vi "harmonic well.vi"() -> ()   [LabVIEW 2019]
uses:
  <vilib>/eio/EIONode/EIONode.xnode
  <vilib>/rvi/eio/common/nirviEmuTemplateMethod_errors.vi
  <vilib>/rvi/DataTransferAndStorage/Container/XNode/niFpgaContainer.xnode
  <vilib>/rvi/FIFO/Fifo_Resource/nirvififoEmulationRead.vi
  <vilib>/eio/EIOPropertyNode/EIOPropertyNode.xnode
  <vilib>/rvi/eio/common/nirviEmuTemplatePropertyGet_errors.vi
  <vilib>/rvi/eio/common/nirviEmuTemplatePropertyGet_noerrors.vi
  <vilib>/rvi/eio/common/nirviEmuTemplatePropertySet_errors.vi
  <vilib>/rvi/eio/common/nirviEmuTemplatePropertySet_noerrors.vi
  <vilib>/rvi/FIFO/Fifo_Resource/nirvififoEmulationWrite.vi
  <vilib>/rvi/interface/RandomDataEmulation/nirviRandomDataFpgaReadWriteTemplate.vi
panel:
  in  "1/Ycali":sgl
  out "Fy out/Ycorr":sgl
  in  "MobY(px/V)":sgl
  in  "Ymean":sgl
  in  "DY":sgl
  in  "Feedback parameters Y":T1
  in  "Enum":enum8{"No FB", "FB"}(ring)
  in  "MobX(px/V)":sgl
  in  "1/Xcali":sgl
  in  "Feedback parameters":T1
  in  "DX":sgl
  in  "Xmean":sgl
  in  "Frequency":u32=100000
  in  "Triangle wave":T2={"signal offset_X"=5.0, "Scale X"=0.0, "signal offset_Y"=5.0, "Scale Y"=0.0, "Phase Shift"=30}
  out "Fx out/Xcorr":sgl
  in  "Xoffset":sgl
  in  "Yoffset":sgl
  in  "sum_offset":sgl
  in  "Normalize signal":bool=TRUE
  in  "FB Time":u8=5 caption="Feedback loop time"
  out "Saveloop":u32
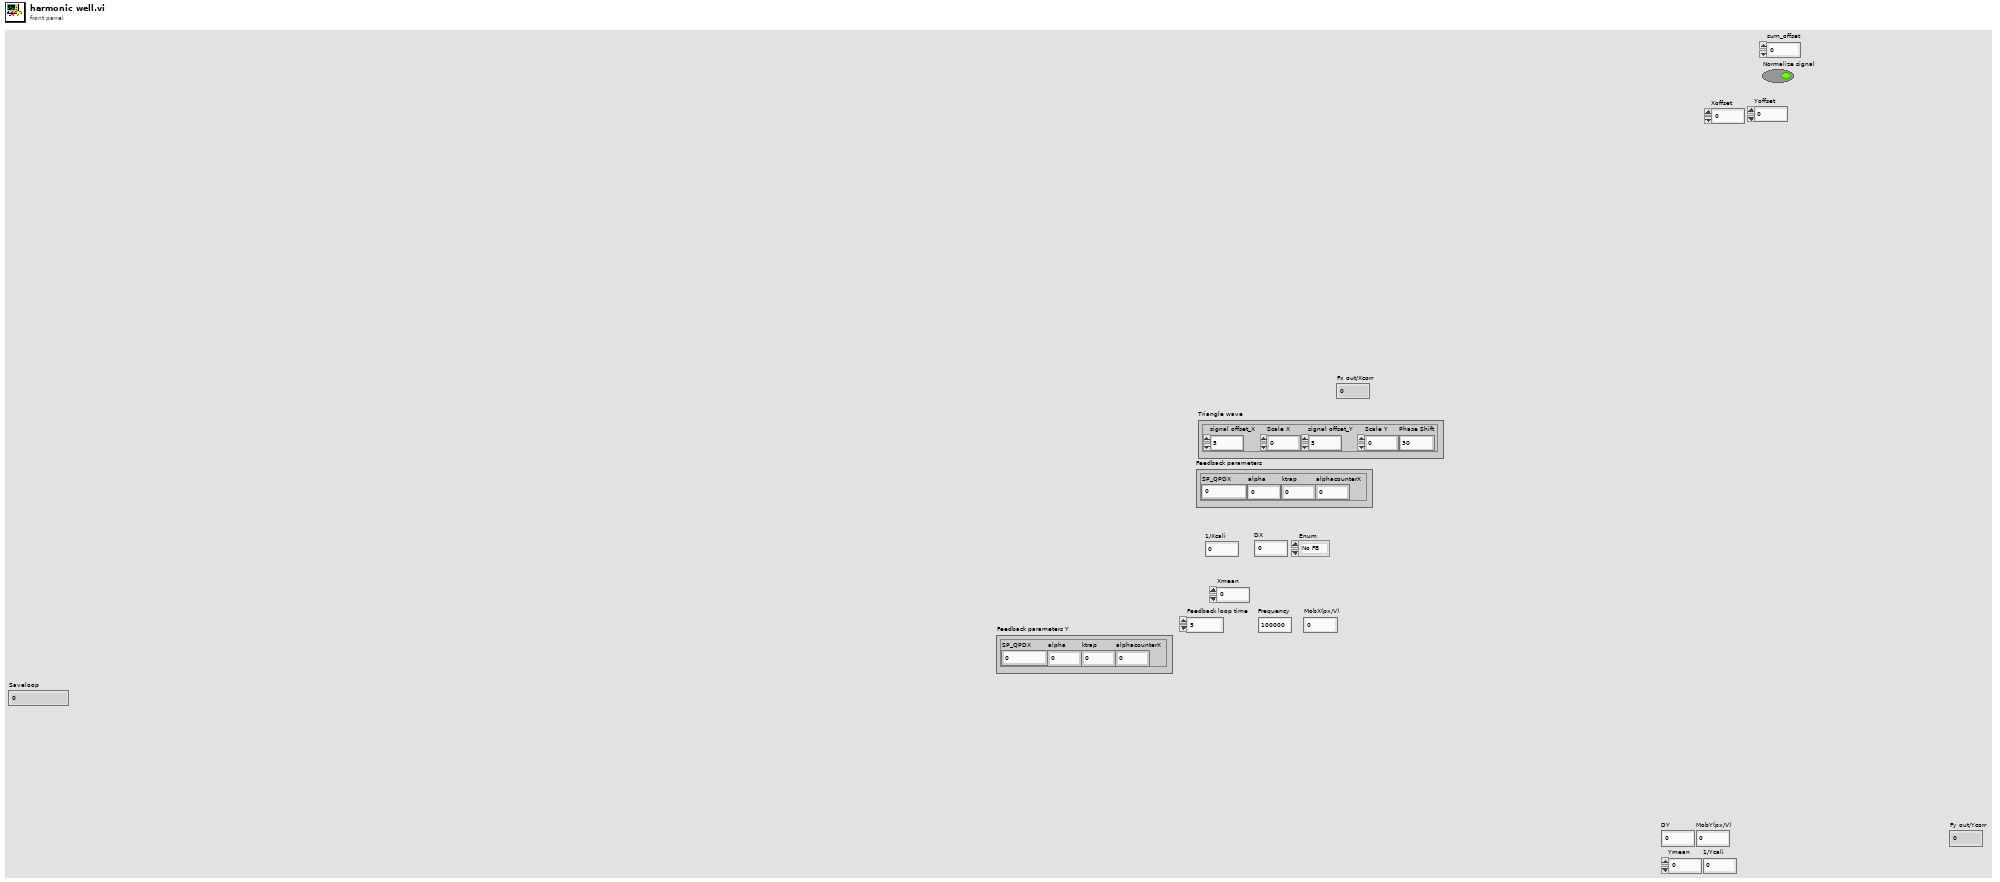
[diagram p1: front panel]
types:
  T1 = cluster{"SP_QPDX":sgl, "alpha":sgl, "ktrap":sgl, "alphacounterX":sgl}
  T2 = cluster{"signal offset_X":sgl, "Scale X":sgl, "signal offset_Y":sgl, "Scale Y":sgl, "Phase Shift":u32}
  T3 = enum8{"+/- 10 V", "+/- 5 V", "+/- 2 V", "+/- 1 V"}
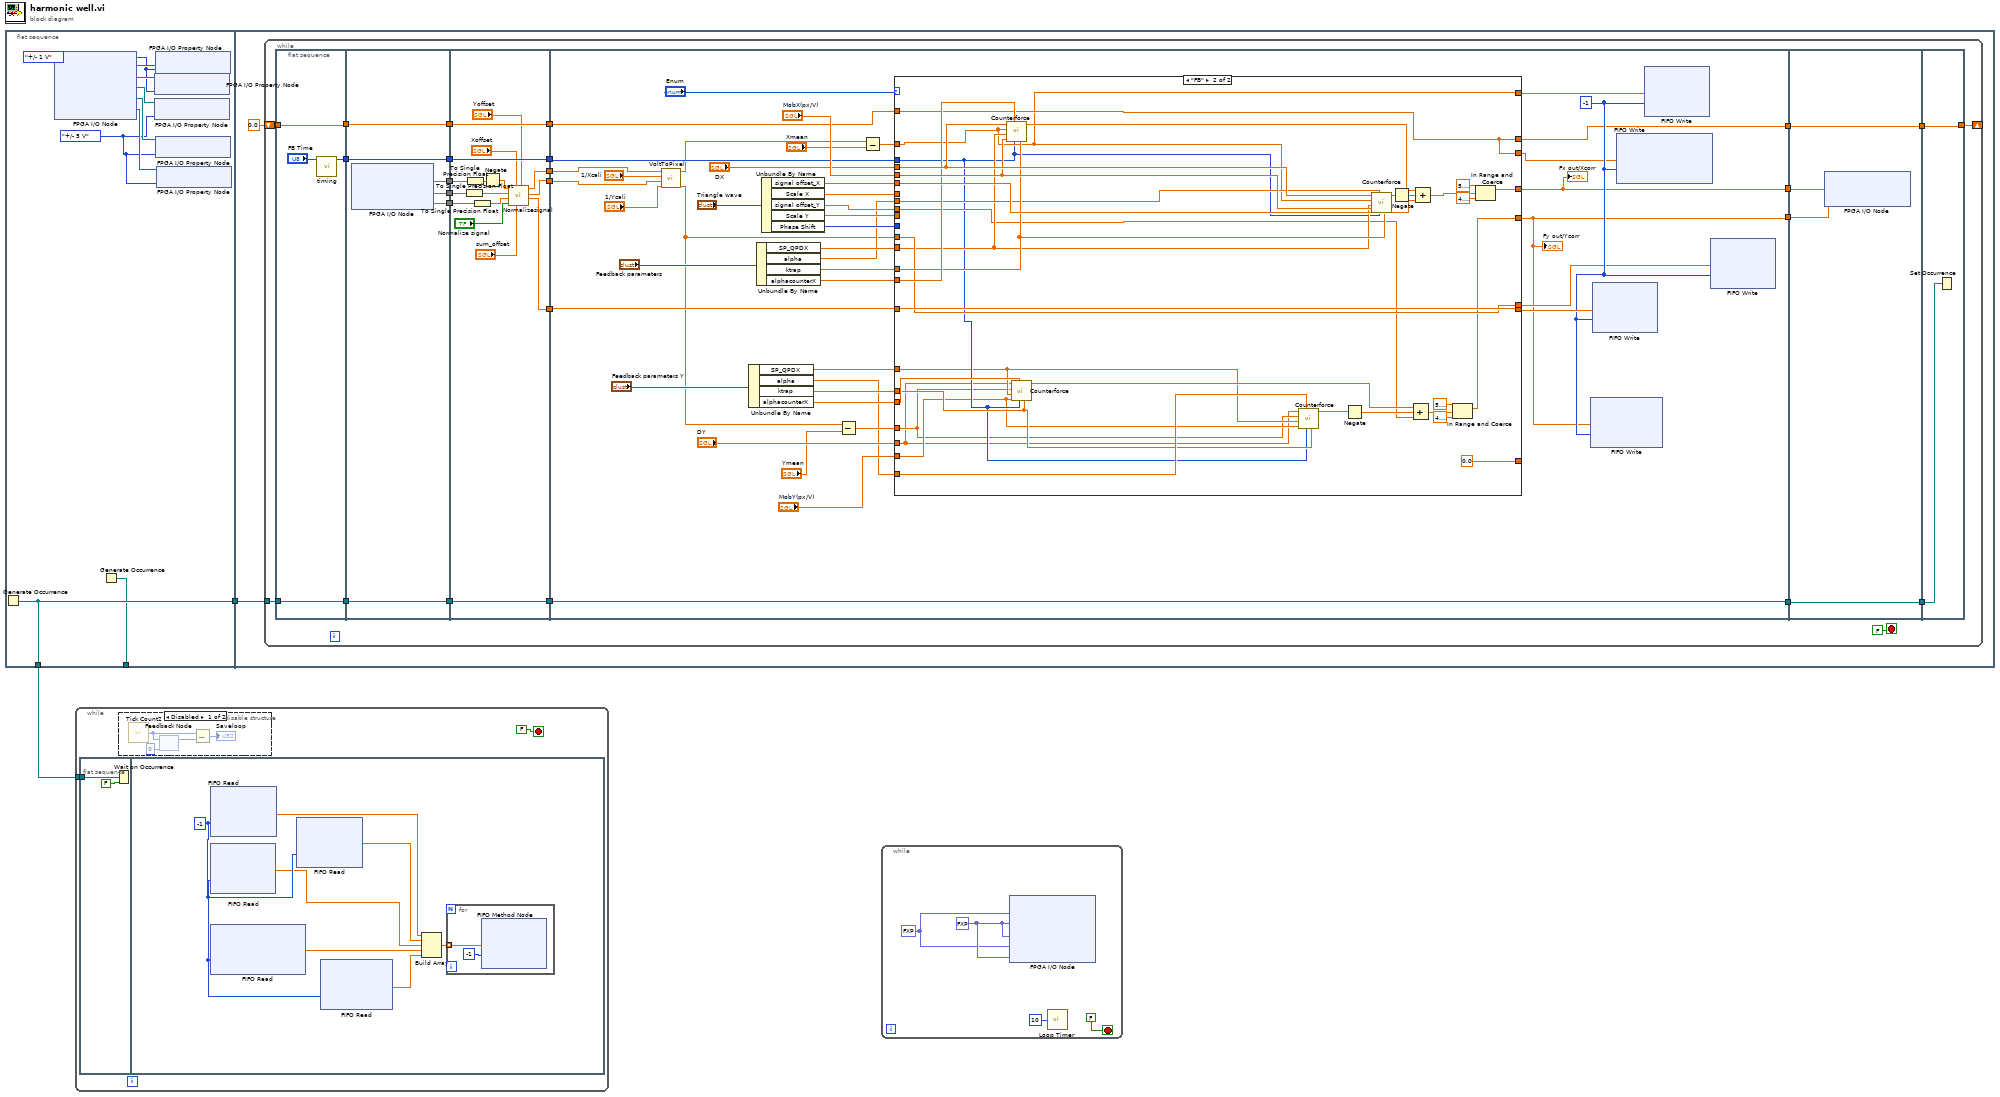
[diagram p0: block diagram]
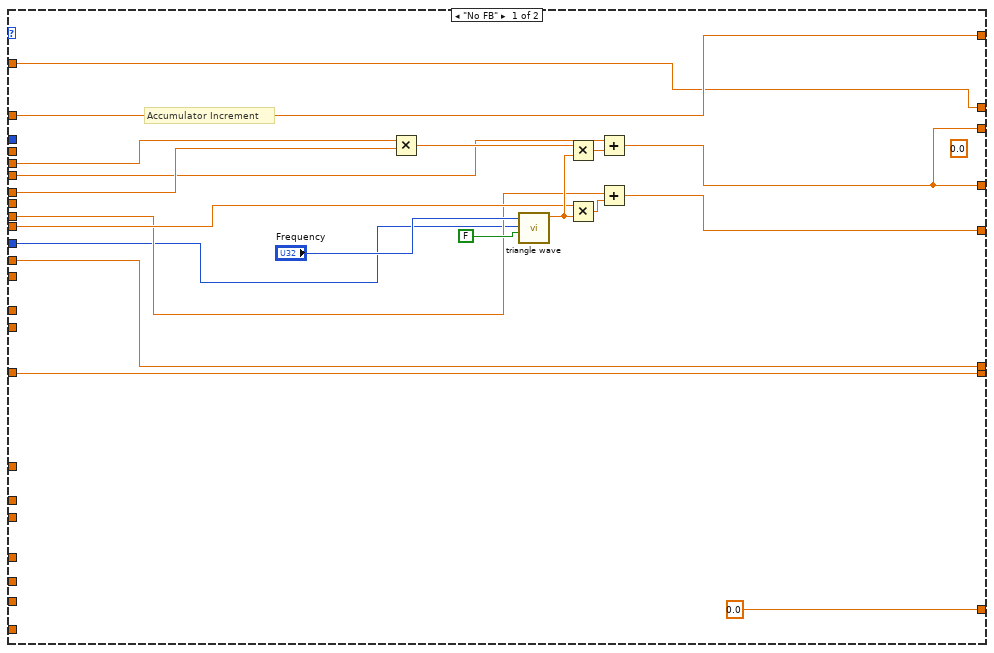
[diagram p2: hidden frame]
diagram:
  n1 = flat-sequence {
    tunnel: [w4] -> w2
    tunnel: [w4] -> w1
    tunnel: [w3] -> _
    tunnel: w2 -> [w13]
    frame #0 {
      w5 = T3."+/- 5 V" ("Voltage Range")
      w8 = T3."+/- 1 V" ("Voltage Range")
      n2 = Generate Occurrence() -> (w4:refnum<k4>)
      n3 = xnode "FPGA I/O Node"() -> ("FPGA I/O Out"=w11:refnum<k21>, "FPGA I/O Out"=w9:refnum<k21>, "FPGA I/O Out"=w10:refnum<k21>, "FPGA I/O Out"=w6:refnum<k21>, "FPGA I/O Out"=w7:refnum<k21>)  [unwired: 5 in, 5 out]
      n4 = Generate Occurrence() -> (w3:refnum<k4>)
      n5 = xnode "FPGA I/O Property Node"("FPGA I/O In"=w9, "Voltage Range"=w8) -> ()  [unwired: 1 out]
      n6 = xnode "FPGA I/O Property Node"("FPGA I/O In"=w10, "Voltage Range"=w5) -> ()  [unwired: 1 out]
      n7 = xnode "FPGA I/O Property Node"("FPGA I/O In"=w11, "Voltage Range"=w8) -> ()  [unwired: 1 out]
      n8 = xnode "FPGA I/O Property Node"("FPGA I/O In"=w6, "Voltage Range"=w5) -> ()  [unwired: 1 out]
      n9 = xnode "FPGA I/O Property Node"("FPGA I/O In"=w7, "Voltage Range"=w5) -> ()  [unwired: 1 out]
    }
    frame #1 {
      n10 = while {
        tunnel: w13 -> [w26]
        shift-right: [w18] -> _
        shift-left: sgl 0.0 -> [w16]
        stop <- FALSE ("stop") stop-if-true
        n11 = flat-sequence {
          tunnel: [w41] -> w27
          tunnel: w26 -> [w40]
          tunnel: [w40] -> w25
          tunnel: [w39] -> w17
          tunnel: w16 -> [w39]
          tunnel: [w48] -> w37
          tunnel: [w47] -> w35
          tunnel: [w46] -> w33
          tunnel: [w45] -> w28
          tunnel: w27 -> [w45]
          tunnel: w25 -> [w44]
          tunnel: [w44] -> w24
          tunnel: w17 -> [w43]
          tunnel: [w43] -> w14
          tunnel: w37 -> [w55]
          tunnel: [w64] -> w36
          tunnel: w35 -> [w54]
          tunnel: [w63] -> w34
          tunnel: w33 -> [w52]
          tunnel: [w62] -> w32
          tunnel: [w65] -> w29
          tunnel: w28 -> [w65]
          tunnel: w24 -> [w61]
          tunnel: [w61] -> w23
          tunnel: [w59] -> w15
          tunnel: w14 -> [w59]
          tunnel: w36 -> [w105]
          tunnel: w34 -> [w74]
          tunnel: w32 -> [w104]
          tunnel: [w80] -> w31
          tunnel: [w67] -> w30
          tunnel: w29 -> [w106]
          tunnel: w23 -> [w99]
          tunnel: [w99] -> w21
          tunnel: [w94] -> w20
          tunnel: w15 -> [w93]
          tunnel: w30 -> [w165]
          tunnel: w31 -> [w166]
          tunnel: [w164] -> w22
          tunnel: w21 -> [w164]
          tunnel: w20 -> [w163]
          tunnel: [w163] -> w19
          tunnel: w22 -> [w168]
          tunnel: [w167] -> w18
          tunnel: w19 -> [w167]
          frame #0 {
            n12 = call "timing.vi"("Feedback loop time"="FB Time") -> ("Feedback Loop time"=w41:u32)  [unwired: 10 in]
          }
          frame #1 {
            n13 = xnode "FPGA I/O Node"() -> ("Connector1/AI2"=w48, "Connector1/AI4"=w47, "Connector1/AI5"=w46)  [unwired: 3 in, 3 out]
          }
          frame #2 {
            n14 = To Single Precision Float(number=w54) -> (single precision float=w53:sgl)
            n15 = To Single Precision Float(number=w55) -> (single precision float=w50:sgl)
            n16 = To Single Precision Float(number=w52) -> (single precision float=w51:sgl)
            n17 = Negate(x=w50) -> (-x=w49:sgl)
            n18 = call "Normalizesignal.vi"("Yoffset"="Yoffset", "sum_offset"="sum_offset", "Xoffset"="Xoffset", "Normalize signal"="Normalize signal", "Sum"=w51, "Y"=w53, "X"=w49) -> ("Sum"=w62:sgl, "Y"=w63:sgl, "X"=w64:sgl)  [unwired: 2 in]
          }
          frame #3 {
            w95 = -1 ("Timeout")
            n19 = call "VoltToPixel.vi"("1/(QPDY/px)"="1/Ycali", "Normalized Y"=w74, "1/(QPDX/px)"="1/Xcali", "Normalized X"=w105) -> ("Ypx"=w66:sgl, "Xpx"=w98:sgl)  [unwired: 6 in]
            n20 = Unbundle By Name("Feedback parameters Y") -> ("SP_QPDX"=w72:sgl, "alpha"=w69:sgl, "ktrap"=w70:sgl, "alphacounterX"=w77:sgl)
            n21 = Unbundle By Name("Feedback parameters") -> ("SP_QPDX"=w85:sgl, "alpha"=w82:sgl, "ktrap"=w83:sgl, "alphacounterX"=w84:sgl)
            n22 = Unbundle By Name("Triangle wave") -> ("signal offset_X"=w89:sgl, "Scale X"=w91:sgl, "signal offset_Y"=w88:sgl, "Scale Y"=w90:sgl, "Phase Shift"=w87:u32)
            n23 = Subtract(x=w66, y="Ymean") -> (x-y=w73:sgl)
            n24 = Subtract(x=w98, y="Xmean") -> (x-y=w102:sgl)
            n25 = case shown="\"FB\"" "Enum" {
              tunnel: w102 -> [w125 w144]
              tunnel: [w109 w159] -> w80
              tunnel: [w119 w134] -> w67
              tunnel: [w125 w144] -> w101
              tunnel: [w127 w150] -> w100
              tunnel: w104 -> [w127 w150]
              tunnel: w66 -> [w126 w149]
              tunnel: [w126 w149] -> w81
              tunnel: "MobX(px/V)" -> [w118 w161]
              tunnel: w106 -> [_ w132]
              tunnel: "DX" -> [_ w162]
              tunnel: [sgl 0.0 ("f") sgl 0.0 ("f")] -> _
              tunnel: [w117 w151] -> w94
              tunnel: w93 -> [w117 w151]
              tunnel: w91 -> [w115 _]
              tunnel: w90 -> [w114 _]
              tunnel: w89 -> [w113 w158]
              tunnel: w88 -> [w112 w135]
              tunnel: w87 -> [w111 _]
              tunnel: w85 -> [_ w145]
              tunnel: w84 -> [_ w157]
              tunnel: w83 -> [_ w156]
              tunnel: w82 -> [_ w155]
              tunnel: [w109 w151] -> w79
              tunnel: w77 -> [_ w143]
              tunnel: "DY" -> [_ w128]
              tunnel: w73 -> [_ w129]
              tunnel: w72 -> [_ w130]
              tunnel: "MobY(px/V)" -> [_ w131]
              tunnel: w70 -> [_ w133]
              tunnel: w69 -> [_ w140]
              frame "No FB" {
                (unwired) sgl 0.0 ("f")
                # "Accumulator Increment"
                n26 = Multiply(x=w118, y=w115) -> (x*y=w123:sgl)
                n27 = call "triangle wave.vi"("Reset Accumulator_TW"=FALSE, "phase shift"=w111, "Frequency"="Frequency") -> ("Tri wave out"=w120:sgl)  [unwired: 8 in]
                n28 = Multiply(x=w123, y=w120) -> (x*y=w122:sgl)
                n29 = Multiply(x=w114, y=w120) -> (x*y=w124:sgl)
                n30 = Add(x=w113, y=w122) -> (x+y=w109:sgl)
                n31 = Add(x=w112, y=w124) -> (x+y=w119:sgl)
              }
              frame "FB" {
                n32 = call "Counterforce.vi"("ktrap"=w156, "Ts"=w132, "alphacounterX"=w157, "mobX(px/V)"=w161, "SP_X"=w145, "Xpx"=w144, "Dx"=w162) -> ("counter Force"=w160:sgl)  [unwired: 2 in, 2 out]
                n33 = call "Counterforce.vi"("ktrap"=w133, "Ts"=w132, "alphacounterX"=w143, "mobX(px/V)"=w131, "SP_X"=w130, "Xpx"=w129, "Dx"=w128) -> ("counter Force"=w137:sgl)  [unwired: 2 in, 2 out]
                n34 = call "Counterforce.vi"("ktrap"=w133, "Ts"=w132, "alphacounterX"=w140, "mobX(px/V)"=w131, "SP_X"=w130, "Xpx"=w129, "Dx"=w128) -> ("counter Force"=w139:sgl)  [unwired: 2 in, 2 out]
                n35 = Negate(x=w139) -> (-x=w138:sgl)
                n36 = call "Counterforce.vi"("ktrap"=w156, "Ts"=w132, "alphacounterX"=w155, "mobX(px/V)"=w161, "SP_X"=w145, "Xpx"=w144, "Dx"=w162) -> ("counter Force"=w148:sgl)  [unwired: 2 in, 2 out]
                n37 = Negate(x=w148) -> (-x=w147:sgl)
                n38 = Compound Arithmetic op=ADD(w137, w138, w135) -> (w136:sgl)
                n39 = Compound Arithmetic op=ADD(w160, w147, w158) -> (w154:sgl)
                n40 = In Range and Coerce(upper limit=sgl 5.1, x=w136, lower limit=sgl 4.9) -> (coerced(x)=w134:sgl)  [unwired: 1 out]
                n41 = In Range and Coerce(upper limit=sgl 5.1, x=w154, lower limit=sgl 4.9) -> (coerced(x)=w159:sgl)  [unwired: 1 out]
              }
            }
            "Fx out/Xcorr" <- w80
            "Fy out/Ycorr" <- w67
            n42 = xnode ("FIFO Write")("Element"=w67, "Timeout"=w95) -> ()  [unwired: 1 in, 2 out]
            n43 = xnode ("FIFO Write")("Element"=w100, "Timeout"=w95) -> ()  [unwired: 1 in, 2 out]
            n44 = xnode ("FIFO Write")("Element"=w79, "Timeout"=w95) -> ()  [unwired: 1 in, 2 out]
            n45 = xnode ("FIFO Write")("Element"=w101, "Timeout"=w95) -> ()  [unwired: 1 in, 2 out]
            n46 = xnode ("FIFO Write")("Element"=w81, "Timeout"=w95) -> ()  [unwired: 1 in, 2 out]
          }
          frame #4 {
            n47 = xnode "FPGA I/O Node"("Connector1/AO7"=w166, "Connector1/AO6"=w165) -> ()  [unwired: 2 in, 2 out]
          }
          frame #5 {
            n48 = Set Occurrence(w168) -> ()
          }
        }
      }
    }
  }
  n49 = while {
    tunnel: w1 -> [w169]
    stop <- FALSE stop-if-true
    n50 = flat-sequence {
      tunnel: w169 -> [w176]
      frame #0 {
        n51 = Wait on Occurrence(1:FALSE ("ignore previous (T)"), 2:w176) -> ()  [unwired: 1 in, 1 out]
      }
      frame #1 {
        w179 = -1 ("Timeout")
        n52 = xnode ("FIFO Read")("Timeout"=w179) -> ("Element"=w177:sgl)  [unwired: 1 in, 2 out]
        n53 = xnode ("FIFO Read")("Timeout"=w179) -> ("Element"=w180:sgl)  [unwired: 1 in, 2 out]
        n54 = xnode ("FIFO Read")("Timeout"=w179) -> ("Element"=w181:sgl)  [unwired: 1 in, 2 out]
        n55 = xnode ("FIFO Read")("Timeout"=w179) -> ("Element"=w178:sgl)  [unwired: 1 in, 2 out]
        n56 = xnode ("FIFO Read")("Timeout"=w179) -> ("Element"=w182:sgl)  [unwired: 1 in, 2 out]
        n57 = Build Array(w181, w178, w177, w180, w182) -> (w183:sgl[])
        n58 = for {
          tunnel: w183 -> [w185] mode=indexing
          n59 = xnode ("FIFO Method Node")("Element"=w185, "Timeout"=-1) -> ()  [unwired: 1 in, 2 out]
        }
      }
    }
    n60 = disable-structure shown="Disabled" {
      frame Disabled {
        n61 = call "Tick Count2"() -> ("Tick Count(uSec)"=w174:u32)
        n62 = feedback #1(u32 0 ("Tick Count(uSec)")) -> (w173:u32)
        n63 = feedback-in #1(w174) -> ()
        n64 = Subtract(x=w174, y=w173) -> (x-y=→"Saveloop":u32)
      }
      frame Enabled {
      }
    }
  }
  n65 = while {
    stop <- FALSE stop-if-true
    w186 = fxp<+,8,3> 2.5 ("Connector1/AO2")
    w187 = fxp<+,8,3> 5.0 ("Connector1/AO2")
    n66 = xnode "FPGA I/O Node"("Connector1/AO0"=w186, "Connector1/AO2"=w187, "Connector1/AO3"=w187, "Connector1/AO4"=w186, "Connector1/AO5"=w187) -> ()  [unwired: 5 in, 5 out]
    n67 = call "Loop Timer"("Count(uSec)"=u8 10) -> ()  [unwired: 1 out]
  }
